vi "Access Privilege_Disbale Controls.vi"(8 "error in (no error)":errorcluster, 10 "Privilege":string, 11 "Boolean Reference":refnum<vi>[](array[refnum])) -> (0 "error out":errorcluster)   [LabVIEW 2023, in "GUI.lvlib"]
uses:
  GUI.lvlib
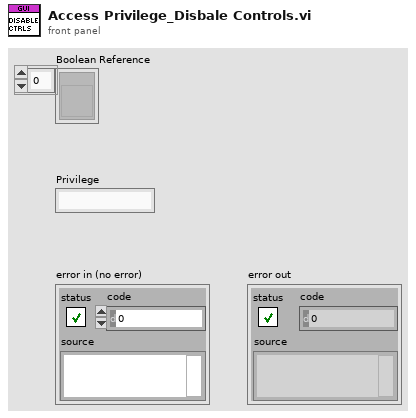
[diagram p1: front panel]
types:
  T1 = enum8{"Enabled", "Disabled", "Disabled and Grayed Out"}
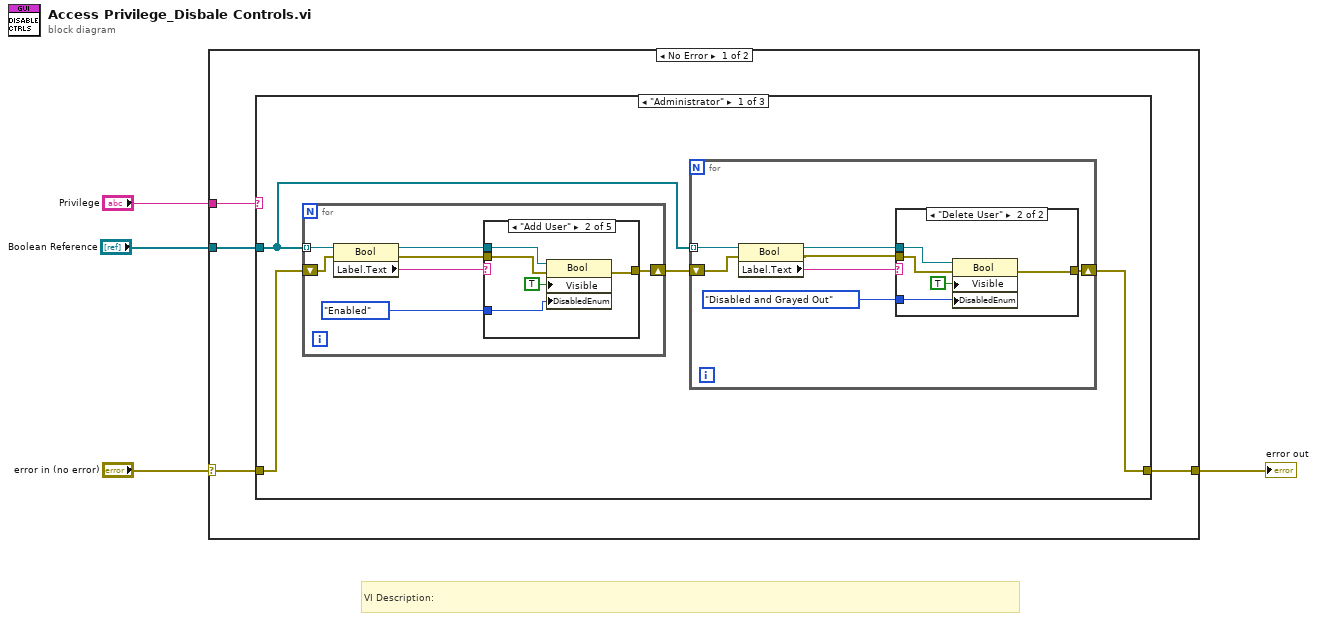
[diagram p0: block diagram]
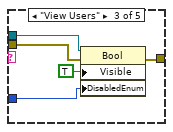
[diagram p4: hidden frame]
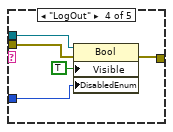
[diagram p5: hidden frame]
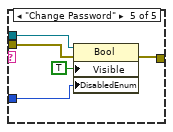
[diagram p6: hidden frame]
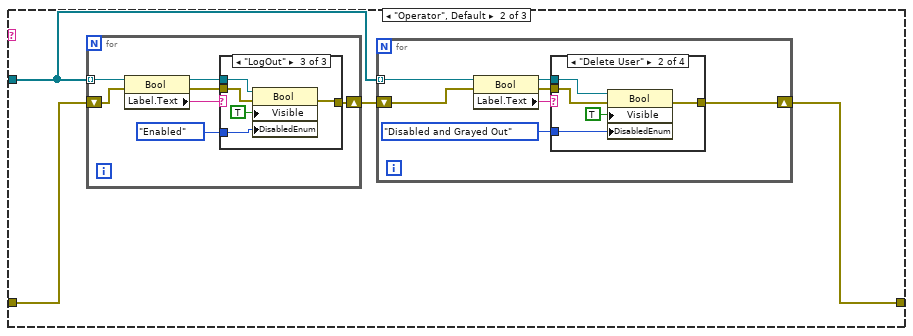
[diagram p7: hidden frame]
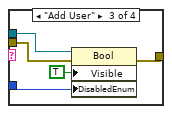
[diagram p9: hidden frame]
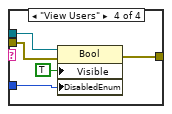
[diagram p10: hidden frame]
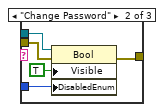
[diagram p12: hidden frame]
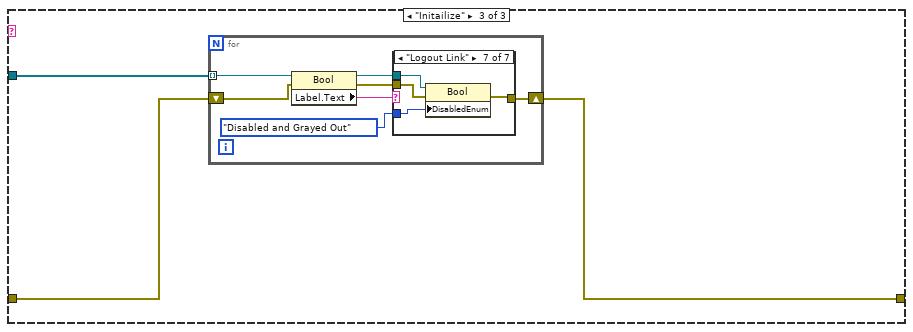
[diagram p13: hidden frame]
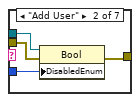
[diagram p15: hidden frame]
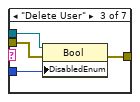
[diagram p16: hidden frame]
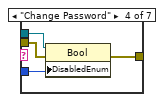
[diagram p17: hidden frame]
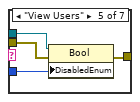
[diagram p18: hidden frame]
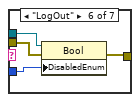
[diagram p19: hidden frame]
diagram:
  # "VI Description:"
  n1 = case shown="No Error" "error in (no error)" {
    selector: "error in (no error)" -> [w8 w134]
    tunnel: [w7 w134] -> w3
    tunnel: "Boolean Reference" -> [w6 _]
    tunnel: "Privilege" -> [w5 _]
    frame No Error {
      n2 = case shown="\"Administrator\"" w5 {
        tunnel: w8 -> [w12 w57 w100]
        tunnel: w6 -> [w11 w56 w101]
        tunnel: [w9 w54 w99] -> w7
        frame "Administrator" {
          n3 = for {
            shift-right: [w30] -> w10
            shift-left: w12 -> [w31]
            tunnel: w11 -> [w28] mode=indexing
            n4 = property class="Bool"(reference=w28, error in=w31) -> (reference out=w27:refnum<vi>, error out=w26:errorcluster, "Label.Text"=w29:string)
            n5 = case shown="\"Add User\"" w29 {
              tunnel: w27 -> [_ w38 w43 w48 w53]
              tunnel: T1."Enabled" ("Disabled") -> [_ w35 w40 w45 w50]
              tunnel: w26 -> [w33 w37 w42 w47 w52]
              tunnel: [w33 w36 w41 w46 w51] -> w30
              frame "False", Default {
              }
              frame "Add User" {
                n6 = property class="Bool"(reference=w38, error in=w37, "Visible"=TRUE, "DisabledEnum"=w35) -> (error out=w36:errorcluster)  [unwired: 1 out]
              }
              frame "View Users" {
                n7 = property class="Bool"(reference=w43, error in=w42, "Visible"=TRUE, "DisabledEnum"=w40) -> (error out=w41:errorcluster)  [unwired: 1 out]
              }
              frame "LogOut" {
                n8 = property class="Bool"(reference=w48, error in=w47, "Visible"=TRUE, "DisabledEnum"=w45) -> (error out=w46:errorcluster)  [unwired: 1 out]
              }
              frame "Change Password" {
                n9 = property class="Bool"(reference=w53, error in=w52, "Visible"=TRUE, "DisabledEnum"=w50) -> (error out=w51:errorcluster)  [unwired: 1 out]
              }
            }
          }
          n10 = for {
            shift-right: [w17] -> w9
            shift-left: w10 -> [w18]
            tunnel: w11 -> [w15] mode=indexing
            n11 = property class="Bool"(reference=w15, error in=w18) -> (reference out=w14:refnum<vi>, error out=w13:errorcluster, "Label.Text"=w16:string)
            n12 = case shown="\"Delete User\"" w16 {
              tunnel: w14 -> [_ w23]
              tunnel: T1."Disabled and Grayed Out" ("Disabled") -> [_ w22]
              tunnel: w13 -> [w20 w24]
              tunnel: [w20 w25] -> w17
              frame "False", Default {
              }
              frame "Delete User" {
                n13 = property class="Bool"(reference=w23, error in=w24, "Visible"=TRUE, "DisabledEnum"=w22) -> (error out=w25:errorcluster)  [unwired: 1 out]
              }
            }
          }
        }
        frame "Operator", Default {
          n14 = for {
            shift-right: [w83] -> w55
            shift-left: w57 -> [w85]
            tunnel: w56 -> [w81] mode=indexing
            n15 = property class="Bool"(reference=w81, error in=w85) -> (reference out=w87:refnum<vi>, error out=w84:errorcluster, "Label.Text"=w82:string)
            n16 = case shown="\"LogOut\"" w82 {
              tunnel: w87 -> [_ w93 w98]
              tunnel: T1."Enabled" ("Disabled") -> [_ w90 w95]
              tunnel: w84 -> [w88 w92 w97]
              tunnel: [w88 w91 w96] -> w83
              frame "False", Default {
              }
              frame "Change Password" {
                n17 = property class="Bool"(reference=w93, error in=w92, "Visible"=TRUE, "DisabledEnum"=w90) -> (error out=w91:errorcluster)  [unwired: 1 out]
              }
              frame "LogOut" {
                n18 = property class="Bool"(reference=w98, error in=w97, "Visible"=TRUE, "DisabledEnum"=w95) -> (error out=w96:errorcluster)  [unwired: 1 out]
              }
            }
          }
          n19 = for {
            shift-right: [w60] -> w54
            shift-left: w55 -> [w62]
            tunnel: w56 -> [w58] mode=indexing
            n20 = property class="Bool"(reference=w58, error in=w62) -> (reference out=w64:refnum<vi>, error out=w61:errorcluster, "Label.Text"=w59:string)
            n21 = case shown="\"Delete User\"" w59 {
              tunnel: w64 -> [_ w68 w73 w79]
              tunnel: T1."Disabled and Grayed Out" ("Disabled") -> [_ w66 w72 w77]
              tunnel: w61 -> [w65 w69 w74 w80]
              tunnel: [w65 w70 w75 w78] -> w60
              frame "False", Default {
              }
              frame "Delete User" {
                n22 = property class="Bool"(reference=w68, error in=w69, "Visible"=TRUE, "DisabledEnum"=w66) -> (error out=w70:errorcluster)  [unwired: 1 out]
              }
              frame "Add User" {
                n23 = property class="Bool"(reference=w73, error in=w74, "Visible"=TRUE, "DisabledEnum"=w72) -> (error out=w75:errorcluster)  [unwired: 1 out]
              }
              frame "View Users" {
                n24 = property class="Bool"(reference=w79, error in=w80, "Visible"=TRUE, "DisabledEnum"=w77) -> (error out=w78:errorcluster)  [unwired: 1 out]
              }
            }
          }
        }
        frame "Initailize" {
          n25 = for {
            shift-right: [w104] -> w99
            shift-left: w100 -> [w106]
            tunnel: w101 -> [w102] mode=indexing
            n26 = property class="Bool"(reference=w102, error in=w106) -> (reference out=w108:refnum<vi>, error out=w105:errorcluster, "Label.Text"=w103:string)
            n27 = case shown="\"Logout Link\"" w103 {
              tunnel: w108 -> [_ w113 w116 w120 w124 w128 w132]
              tunnel: T1."Disabled and Grayed Out" ("Disabled") -> [_ w112 w117 w121 w125 w129 w133]
              tunnel: w105 -> [w109 w111 w115 w118 w123 w127 w131]
              tunnel: [w109 w110 w114 w119 w122 w126 w130] -> w104
              frame "False", Default {
              }
              frame "Add User" {
                n28 = property class="Bool"(reference=w113, error in=w111, "DisabledEnum"=w112) -> (error out=w110:errorcluster)  [unwired: 1 out]
              }
              frame "Delete User" {
                n29 = property class="Bool"(reference=w116, error in=w115, "DisabledEnum"=w117) -> (error out=w114:errorcluster)  [unwired: 1 out]
              }
              frame "Change Password" {
                n30 = property class="Bool"(reference=w120, error in=w118, "DisabledEnum"=w121) -> (error out=w119:errorcluster)  [unwired: 1 out]
              }
              frame "View Users" {
                n31 = property class="Bool"(reference=w124, error in=w123, "DisabledEnum"=w125) -> (error out=w122:errorcluster)  [unwired: 1 out]
              }
              frame "LogOut" {
                n32 = property class="Bool"(reference=w128, error in=w127, "DisabledEnum"=w129) -> (error out=w126:errorcluster)  [unwired: 1 out]
              }
              frame "Logout Link" {
                n33 = property class="Bool"(reference=w132, error in=w131, "DisabledEnum"=w133) -> (error out=w130:errorcluster)  [unwired: 1 out]
              }
            }
          }
        }
      }
    }
    frame Error {
    }
  }
  "error out" <- w3
